vi "TestExec.Read Config for Executable and Args.vi"(8 "error in":errorcluster, 10 "Vars":variant, 11 "Config File":path) -> (0 "error out":errorcluster, 1 "Args":string[](array[string]), 2 "Exe":path, 3 "Action Name":string, 4 "Error Code":i32, 5 "Data Name Prefix":string, 6 "IgnoreStdError":bool, 7 "OutType":i32)   [LabVIEW 2024]
uses:
  <vilib>/Utility/config.llb/Config Data RefNum.ctl
  Errors/Error.Error Code List.ctl
  <vilib>/Utility/config.llb/Read Key (Path).vi
  <vilib>/Utility/config.llb/Read Key (String).vi
  <vilib>/Utility/config.llb/Read Key (I32).vi
  <vilib>/Utility/config.llb/Read Key (Boolean).vi
  <vilib>/Utility/config.llb/NI_LVConfig.lvlib
  Errors.lvlib
  <vilib>/KATE/Files/File Utils.lvlib
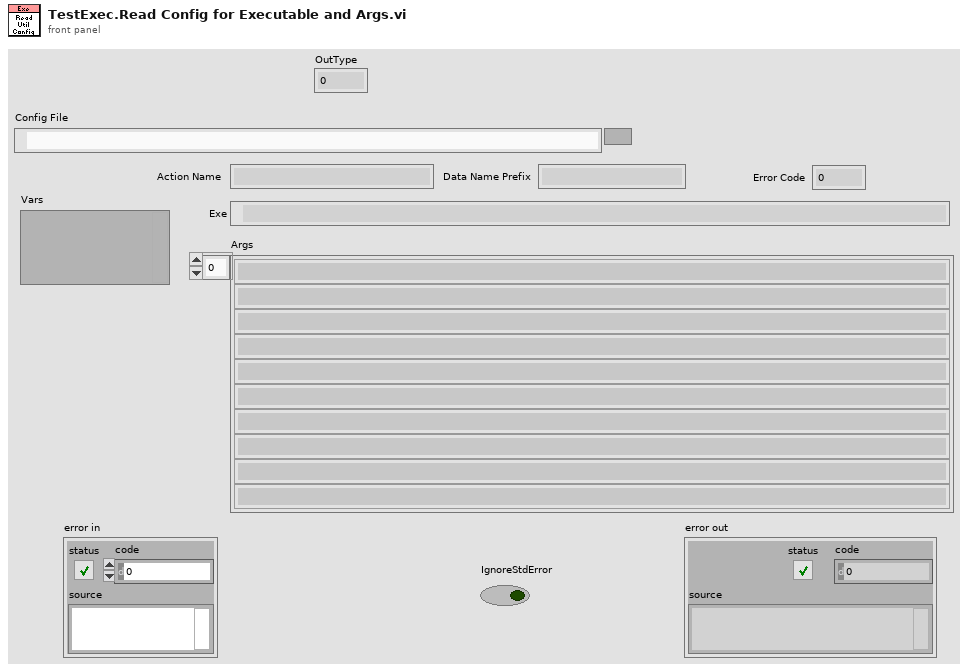
[diagram p1: front panel]
types:
  T1 = typedef "NI_LVConfig.lvlib/Config Data RefNum.ctl" = refnum<k1>
  T2 = cluster{"Exe":path, "Args":string[], "FileRef":T1, "Name":string, "Prefix":string, "Code":i32, "IgnoreStdErr":bool, "CheckExePath":bool, "OutType":i32}
  T3 = typedef "EQMF.lvlib/Errors.lvlib/Error.Error Code List.ctl" = i32
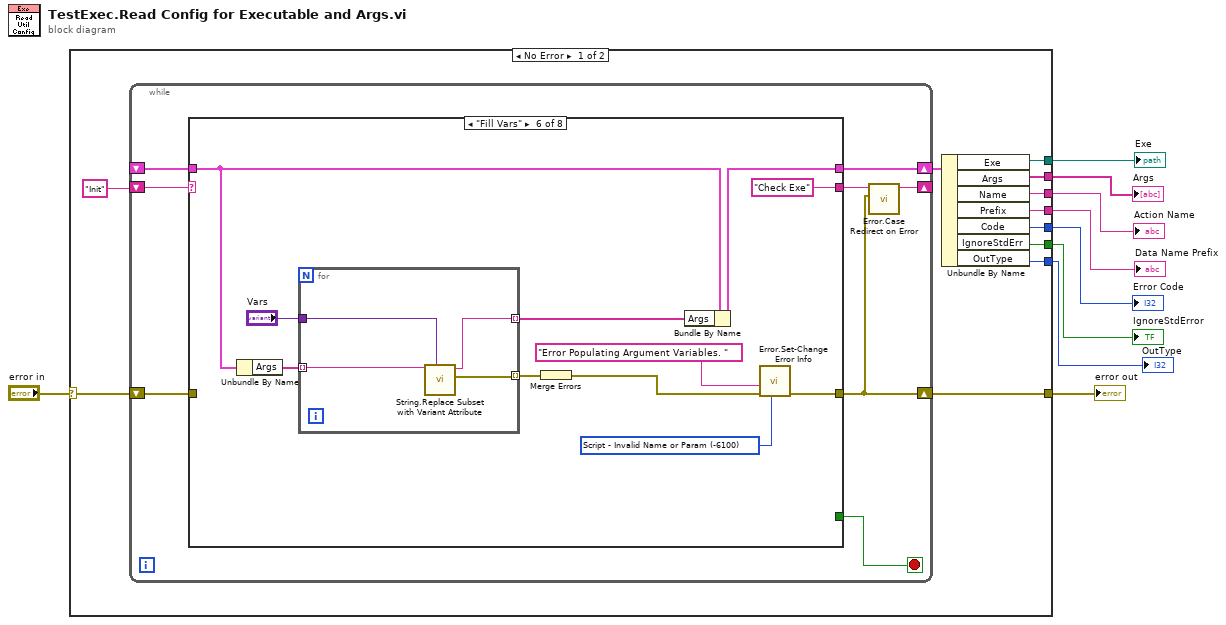
[diagram p0: block diagram]
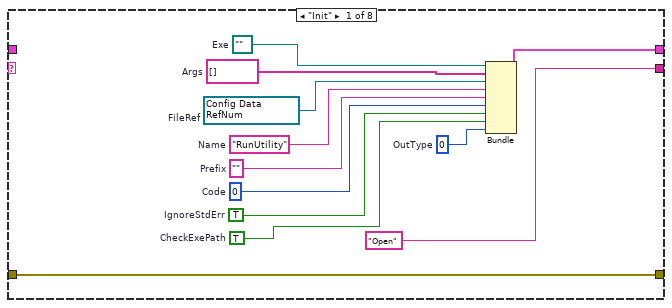
[diagram p2: hidden frame]
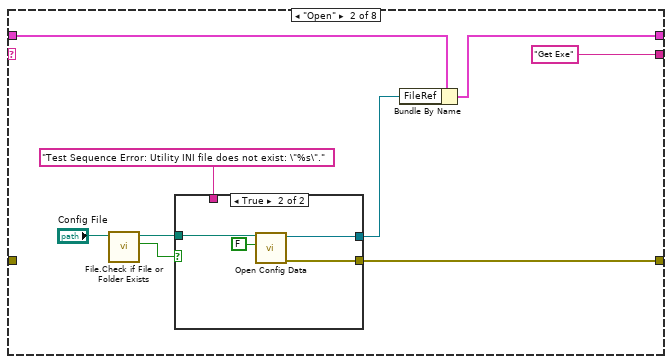
[diagram p3: hidden frame]
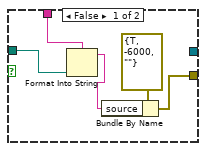
[diagram p4: hidden frame]
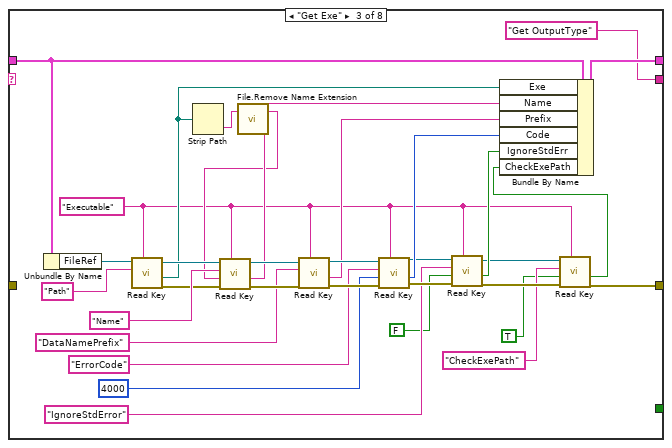
[diagram p5: hidden frame]
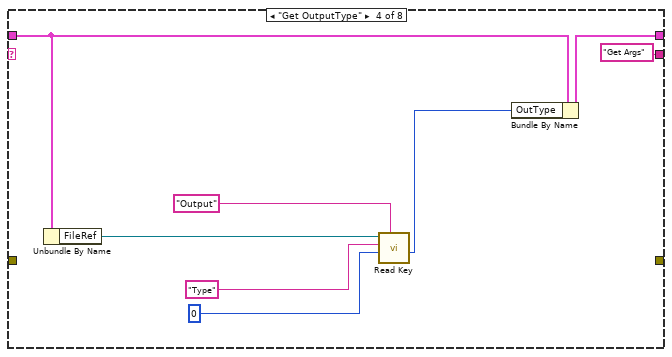
[diagram p6: hidden frame]
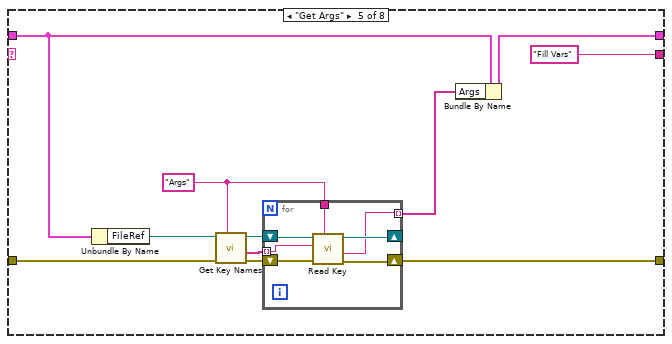
[diagram p7: hidden frame]
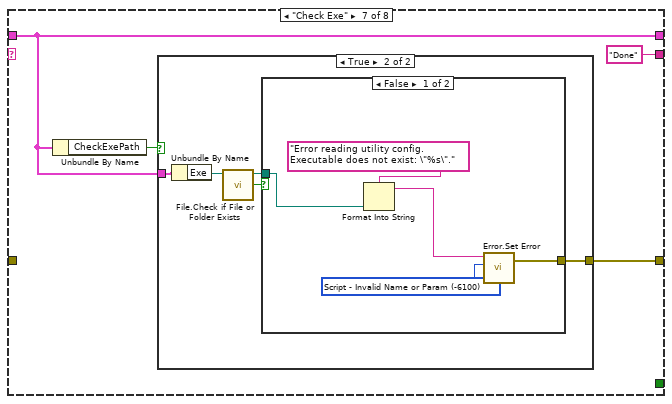
[diagram p8: hidden frame]
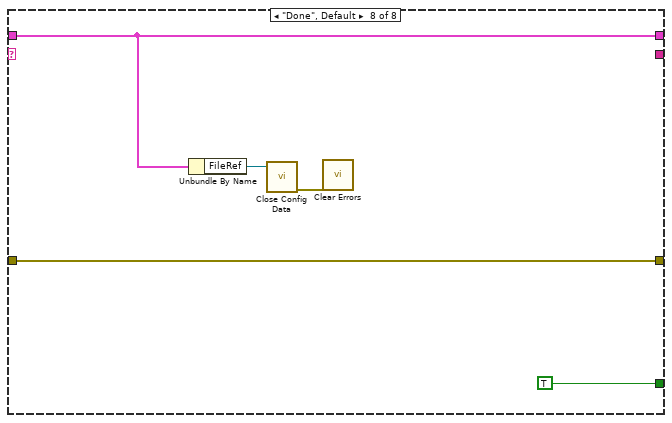
[diagram p11: hidden frame]
diagram:
  n1 = case shown="No Error" "error in" {
    selector: "error in" -> [w19 w152]
    tunnel: [w16 _] -> w6
    tunnel: [w15 _] -> w9
    tunnel: [w18 w152] -> w8
    tunnel: [w14 _] -> w5
    tunnel: [w13 _] -> w4
    tunnel: [w12 _] -> w3
    tunnel: [w11 _] -> w2
    tunnel: [w10 _] -> w1
    frame No Error {
      n2 = while {
        shift-right: [w26] -> w17
        shift-left: _ -> [w27]
        shift-right: [w25] -> _
        shift-left: "Init" -> [w28]
        shift-right: [w22] -> w18
        shift-left: w19 -> [w23]
        stop <- w21 stop-if-true
        n3 = case shown="\"Fill Vars\"" w28 {
          tunnel: w27 -> [_ w46 w90 w98 w103 w118 w134 w150]
          tunnel: [w37 w47 w91 w99 w104 w125 w134 w150] -> w26
          tunnel: ["Open" ("String") "Get Exe" ("String") "Get OutputType" ("String") "Get Args" ("String") "Fill Vars" ("String") "Check Exe" ("String") "Done" ("String") _] -> w24
          tunnel: w23 -> [w35 _ _ _ w106 _ _ w147]
          tunnel: [w35 w49 w65 _ w105 w123 w135 w147] -> w22
          tunnel: [_ _ _ _ _ _ _ TRUE] -> w21
          frame "Init" {
            w29 = 0  # OutType
            w30 = TRUE  # CheckExePath
            w31 = TRUE  # IgnoreStdErr
            w34 = "RunUtility"  # Name
            w32 = 0  # Code
            w33 = ""  # Prefix
            w38 = T1 refnum items=["config data"]  # FileRef
            w40 = path ""  # Exe
            w39 = string[] []  # Args
            n4 = Bundle("Exe"=w40, "Args"=w39, "FileRef"=w38, "Name"=w34, "Prefix"=w33, "Code"=w32, "IgnoreStdErr"=w31, "CheckExePath"=w30, "OutType"=w29) -> (w37:T2)  [unwired: 1 in]
          }
          frame "Open" {
            n5 = call <vilib>:"File.Check if File or Folder Exists.vi"("Path"="Config File") -> ("Exists"=w42:bool, "Dup Path"=w43:path)  [unwired: 6 in, 3 out]
            n6 = case shown="True" w42 {
              tunnel: [w53 w58] -> w49
              tunnel: [_ w57] -> w48
              tunnel: w43 -> [w52 w56]
              tunnel: "Test Sequence Error: Utility INI file does not exist: \"%s\"." -> [w51 _]
              frame False {
                n7 = Format Into String(format string=w51, w52) -> (resulting string=w50:string)  [unwired: 2 in, 1 out]
                n8 = Bundle By Name(cluster=errorcluster {"status"=TRUE, "code"=-6000, "source"=""} ("error constant"), "source"=w50) -> (w53:errorcluster)
              }
              frame True {
                n9 = call <vilib>:"Open Config Data.vi"("create file if necessary (T)"=FALSE, "configuration file path"=w56) -> ("error out"=w58:errorcluster, "refnum"=w57:T1)  [unwired: 7 in, 1 out]
              }
            }
            n10 = Bundle By Name(cluster=w46, "FileRef"=w48) -> (w47:T2)
          }
          frame "Get Exe" {
            w60 = "Executable"
            n11 = Unbundle By Name(w90) -> ("FileRef"=w88:T1)
            n12 = call-poly <vilib>:"Read Key.vi"("section"=w60, "key"="Path", "refnum"=w88) -> ("error out"=w77:errorcluster, "value"=w73:path, "refnum out"=w82:T1)  [unwired: 5 in, 1 out]
            n13 = Strip Path(path=w73) -> (name=w72:string)  [unwired: 1 out]
            n14 = call <vilib>:"File.Remove Name Extension.vi"("File Name"=w72) -> ("Name Less Ext"=w71:string)  [unwired: 1 in, 1 out]
            n15 = call-poly <vilib>:"Read Key.vi"("section"=w60, "error in (no error)"=w77, "default value"=w71, "key"="Name", "refnum"=w82) -> ("error out"=w86:errorcluster, "value"=w74:string, "refnum out"=w85:T1)  [unwired: 3 in, 1 out]
            n16 = call-poly <vilib>:"Read Key.vi"("section"=w60, "error in (no error)"=w86, "key"="DataNamePrefix", "refnum"=w85) -> ("error out"=w84:errorcluster, "value"=w80:string, "refnum out"=w83:T1)  [unwired: 4 in, 1 out]
            n17 = call-poly <vilib>:"Read Key.vi"("section"=w60, "error in (no error)"=w84, "default value"=4000, "key"="ErrorCode", "refnum"=w83) -> ("error out"=w69:errorcluster, "value"=w76:i32, "refnum out"=w70:T1)  [unwired: 3 in, 1 out]
            n18 = call-poly <vilib>:"Read Key.vi"("section"=w60, "error in (no error)"=w69, "default value"=FALSE, "key"="IgnoreStdError", "refnum"=w70) -> ("error out"=w64:errorcluster, "value"=w66:bool, "refnum out"=w63:T1)  [unwired: 3 in, 1 out]
            n19 = call-poly <vilib>:"Read Key.vi"("section"=w60, "error in (no error)"=w64, "default value"=TRUE, "key"="CheckExePath", "refnum"=w63) -> ("error out"=w65:errorcluster, "value"=w59:bool)  [unwired: 3 in, 2 out]
            n20 = Bundle By Name(cluster=w90, "Exe"=w73, "Name"=w74, "Prefix"=w80, "Code"=w76, "IgnoreStdErr"=w66, "CheckExePath"=w59) -> (w91:T2)
          }
          frame "Get OutputType" {
            n21 = Unbundle By Name(w98) -> ("FileRef"=w92:T1)
            n22 = call-poly <vilib>:"Read Key.vi"("section"="Output", "default value"=0, "key"="Type", "refnum"=w92) -> ("value"=w95:i32)  [unwired: 4 in, 3 out]
            n23 = Bundle By Name(cluster=w98, "OutType"=w95) -> (w99:T2)
          }
          frame "Get Args" {
            w107 = "Args"
            n24 = Unbundle By Name(w103) -> ("FileRef"=w102:T1)
            n25 = call <vilib>:"Get Key Names.vi"("section"=w107, "error in (no error)"=w106, "refnum"=w102) -> ("error out"=w109:errorcluster, "key names"=w108:string[], "refnum out"=w110:T1)  [unwired: 5 in, 1 out]
            n26 = for {
              tunnel: w107 -> [w117]
              tunnel: w108 -> [w114] mode=indexing
              shift-right: [w113] -> _
              shift-left: w110 -> [w116]
              shift-right: [w112] -> w105
              shift-left: w109 -> [w115]
              tunnel: [w111] -> w101 mode=indexing
              n27 = call-poly <vilib>:"Read Key.vi"("section"=w117, "error in (no error)"=w115, "key"=w114, "refnum"=w116) -> ("error out"=w112:errorcluster, "value"=w111:string, "refnum out"=w113:T1)  [unwired: 4 in, 1 out]
            }
            n28 = Bundle By Name(cluster=w103, "Args"=w101) -> (w104:T2)
          }
          frame "Fill Vars" {
            w121 = T3 -6100 items=["No Error"=0, "Abort"=-2, "Misc"=-5000, "Fixture Error"=-5100, "File IO - General"=-5200, "FIle IO - Config Error"=-5201, "Instrument - General"=-5300, "Instrument - Serial Com"=-5301, "Instrument - Camera"=-5302, "Instrument - PS"=-5303, "Instrument - Oscilloscope"=-5304, "Instrument - Function Gen"=-5305, "Instrument - Load"=-5306, "Instrument - Meter"=-5307, "Instrument - Power Control"=-5308, "Instrument - Motion"=-5309, "Instrument - RF"=-5310, "System Exe"=-5400, "Image Processing"=-5500, "Communication"=-5600, "Script - Syntax Error"=-6000, "Script - Invalid Name or Param"=-6100, "Script - Timeout"=-6200, "Invalid Data"=-6300, "FW Update Error"=-6500] ("Std Code")
            n29 = Unbundle By Name(w118) -> ("Args"=w128:string[])
            n30 = for {
              tunnel: "Vars" -> [w132]
              tunnel: w128 -> [w131] mode=indexing
              tunnel: [w130] -> w127 mode=indexing
              tunnel: [w129] -> w126 mode=indexing
              n31 = call "String.Replace Subset with Variant Attribute.vi"("Vars"=w132, "Data In"=w131) -> ("error out"=w130:errorcluster, "Data Out"=w129:string)  [unwired: 8 in]
            }
            n32 = Merge Errors(w127) -> (w122:errorcluster)
            n33 = Bundle By Name(cluster=w118, "Args"=w126) -> (w125:T2)
            n34 = call "Error.Set-Change Error Info.vi"("Std Code"=w121, "error in"=w122, "Description"="Error Populating Argument Variables. ") -> ("error out"=w123:errorcluster)  [unwired: 8 in]
          }
          frame "Check Exe" {
            n35 = Unbundle By Name(w134) -> ("CheckExePath"=w133:bool)
            n36 = case shown="True" w133 {
              tunnel: w134 -> [_ w141]
              tunnel: [_ w138] -> w135
              frame False {
              }
              frame True {
                n37 = Unbundle By Name(w141) -> ("Exe"=w140:path)
                n38 = call <vilib>:"File.Check if File or Folder Exists.vi"("Path"=w140) -> ("Exists"=w139:bool, "Dup Path"=w137:path)  [unwired: 6 in, 3 out]
                n39 = case shown="False" w139 {
                  tunnel: [w146 _] -> w138
                  tunnel: w137 -> [w143 _]
                  frame False {
                    w145 = T3 -6100 items=["No Error"=0, "Abort"=-2, "Misc"=-5000, "Fixture Error"=-5100, "File IO - General"=-5200, "FIle IO - Config Error"=-5201, "Instrument - General"=-5300, "Instrument - Serial Com"=-5301, "Instrument - Camera"=-5302, "Instrument - PS"=-5303, "Instrument - Oscilloscope"=-5304, "Instrument - Function Gen"=-5305, "Instrument - Load"=-5306, "Instrument - Meter"=-5307, "Instrument - Power Control"=-5308, "Instrument - Motion"=-5309, "Instrument - RF"=-5310, "System Exe"=-5400, "Image Processing"=-5500, "Communication"=-5600, "Script - Syntax Error"=-6000, "Script - Invalid Name or Param"=-6100, "Script - Timeout"=-6200, "Invalid Data"=-6300, "FW Update Error"=-6500] ("Std Code")
                    n40 = Format Into String(format string="Error reading utility config.  Executable does not exist: \"%s\"." ("Desc"), w143) -> (resulting string=w142:string)  [unwired: 2 in, 1 out]
                    n41 = call "Error.Set Error.vi"("Std Code"=w145, "Desc"=w142) -> ("error out"=w146:errorcluster)  [unwired: 5 in]
                  }
                  frame True {
                  }
                }
              }
            }
          }
          frame "Done", Default {
            n42 = Unbundle By Name(w150) -> ("FileRef"=w149:T1)
            n43 = call <vilib>:"Close Config Data.vi"("refnum"=w149) -> ("error out"=w148:errorcluster)  [unwired: 9 in, 1 out]
            n44 = call <vilib>:"Clear Errors.vi"("error in (no error)"=w148) -> ()  [unwired: 5 in, 2 out]
          }
        }
        n45 = call "Error.Case Redirect on Error.vi"("error in"=w22, "Next Case"=w24) -> ("Next Case Out"=w25:string)  [unwired: 9 in]
      }
      n46 = Unbundle By Name(w17) -> ("Exe"=w16:path, "Args"=w15:string[], "Name"=w14:string, "Prefix"=w13:string, "Code"=w12:i32, "IgnoreStdErr"=w11:bool, "OutType"=w10:i32)
    }
    frame Error {
    }
  }
  "Exe" <- w6
  "Args" <- w9
  "error out" <- w8
  "Action Name" <- w5
  "Data Name Prefix" <- w4
  "Error Code" <- w3
  "IgnoreStdError" <- w2
  "OutType" <- w1
